vi "c_ctre_phoenix6_orchestra_GetCurrentTime.vi"(0 "Numeric 2":u16, 1 "Numeric 4":dbl) -> (20 "Numeric":i32, 21 "Numeric 3":dbl)   [LabVIEW 2023]
uses:
  <vilib>/Rock Robotics/WPI/ThirdParty/Phoenix-LabVIEW/Controls/DriverLib.ctl
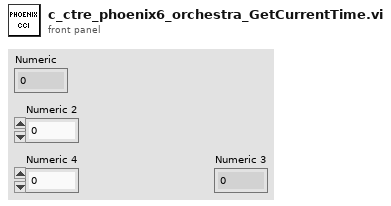
[diagram p1: front panel]
types:
  T1 = typedef "DriverLib.ctl" = path
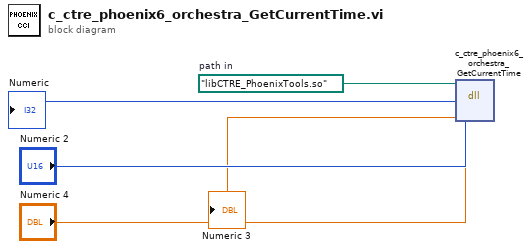
[diagram p0: block diagram]
diagram:
  w5 = T1 path "libCTRE_PhoenixTools.so"  # path in
  n1 = dll-call lib="?" fn="c_ctre_phoenix6_orchestra_GetCurrentTime"(path in=w5, "Numeric 2", "Numeric 4") -> (→"Numeric":i32, →"Numeric 3":dbl)  [unwired: 3 in, 2 out]
